vi "convert GEECS tdms to png.vi"(8 "error in (no error)":errorcluster, 11 "Save Image Path":path) -> (0 "error out":errorcluster)   [LabVIEW 2020, in "Point Grey Camera.lvclass"]
uses:
  Point Grey Camera.lvclass
panel:
  # "reentrant"
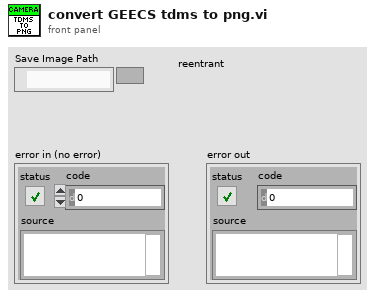
[diagram p1: front panel]
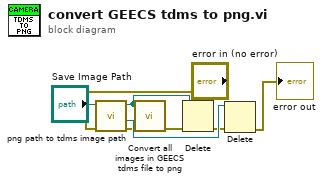
[diagram p0: block diagram]
diagram:
  n1 = call "png path to tdms image path.vi"("error in (no error)"="error in (no error)", "png path"="Save Image Path") -> ("error out"=w2:errorcluster, "tdms index path"=w7:path, "tdms image path"=w5:path)  [unwired: 6 in, 1 out]
  n2 = call "Convert all images in GEECS tdms file to png.vi"("error in (no error)"=w2, "file path"=w5) -> ("error out"=w3:errorcluster)  [unwired: 8 in, 1 out]
  n3 = Delete(path (use dialog)=w5, error in=w3) -> (error out=w6:errorcluster)  [unwired: 3 in, 2 out]
  n4 = Delete(path (use dialog)=w7, error in=w6) -> (error out=→"error out":errorcluster)  [unwired: 3 in, 2 out]
